vi "LossyEnqueueMessage.vi"(8 "error in":errorcluster, 9 "Message Priority (0)":i32, 10 "Message":refnum<class "Message.lvclass">, 11 "PriorityMessageQueue in":refnum<class "PriorityMessageQueue.lvclass">) -> (0 "error out":errorcluster, 1 "Overflow?":bool, 2 "Overflow Message":refnum<class "Message.lvclass">, 3 "PriorityMessageQueue out":refnum<class "PriorityMessageQueue.lvclass">)   [LabVIEW 2009, in "LapDog.Messaging.v2.lvlib" / "PriorityMessageQueue.lvclass"]
doc: "<b>This class is deprecated in version 2.1 and will be removed in version 3.0</b>\n\nAdds a message to the queue with the given priority. If the number of messages at that priority level is equal to the Max Queue Size when the queue was created, the first element with that priority is removed from the queue and discarded."
uses:
  PriorityMessageQueue.lvclass
  MessageObject/Message.lvclass
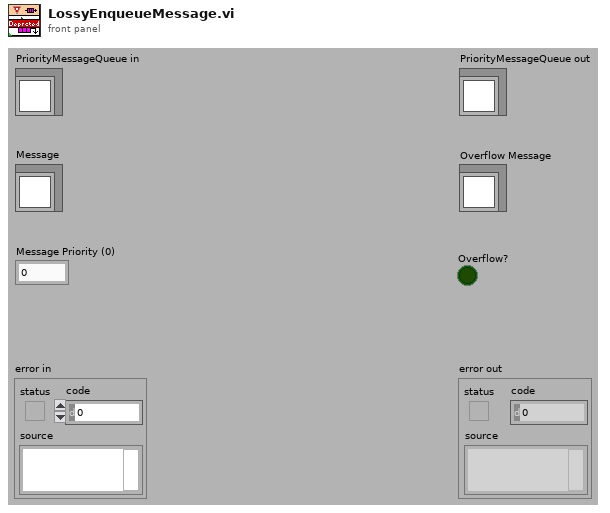
[diagram p1: front panel]
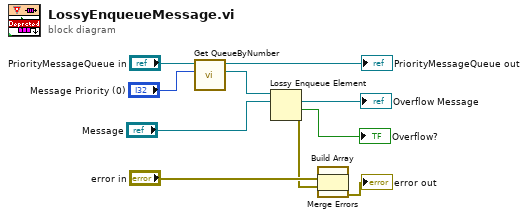
[diagram p0: block diagram]
diagram:
  n1 = call "Get QueueByNumber.vi"("Priority Level"="Message Priority (0)", "PriorityMessageQueue in"="PriorityMessageQueue in") -> ("Message Queue"=w3:refnum<queue>, "PriorityMessageQueue out"=→"PriorityMessageQueue out":refnum<class "PriorityMessageQueue.lvclass">)  [unwired: 8 in]
  n2 = Lossy Enqueue Element(queue=w3, element="Message") -> (overflow element=→"Overflow Message":refnum<class "Message.lvclass">, overflow?=→"Overflow?":bool, error out=w6:errorcluster)  [unwired: 1 in, 1 out]
  n3 = Build Array("error in", w6) -> (w1:errorcluster[])
  n4 = call <vilib>:"Merge Errors.vi"("error array in"=w1) -> ("error out"=→"error out":errorcluster)  [unwired: 6 in]
